vi "FTW-JSON-Serialize.vi"(0 "JSON Object":refnum<class "FTW-JSON.lvclass">, 11 "error in":errorcluster) -> (4 "JSON Object out":refnum<class "FTW-JSON.lvclass">, 6 "JSON String (UTF-8)":string, 15 "error out":errorcluster)   [LabVIEW 2012, in "FTW-JSON.lvclass"]
uses:
  FTW-JSON.lvclass
  FTW-JSON.lvclass/FTW-JSON.ctl
panel:
  # "Inputs"
  # "Outputs"
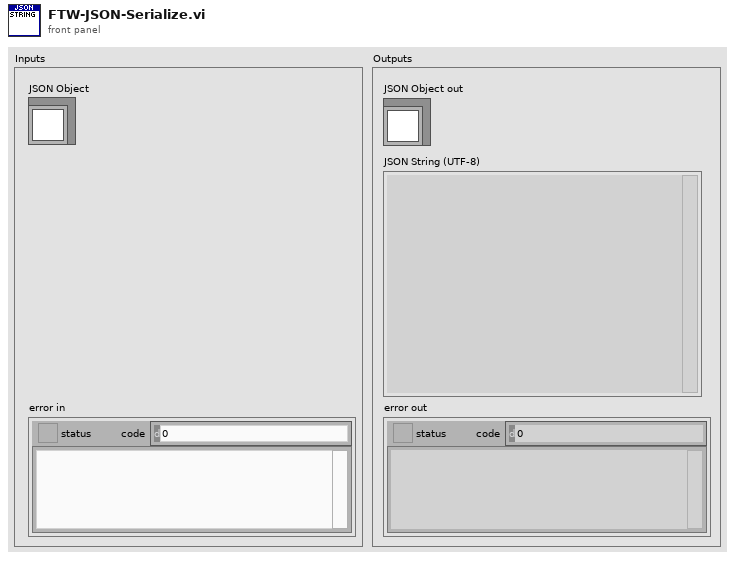
[diagram p1: front panel]
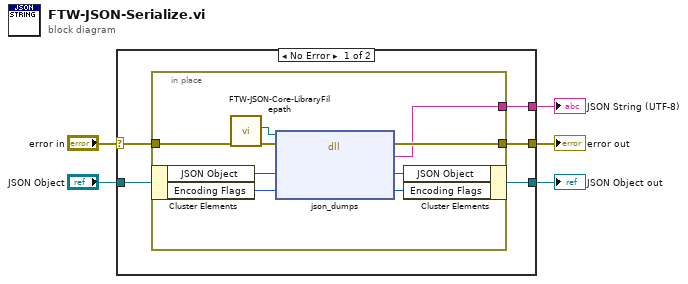
[diagram p0: block diagram]
diagram:
  n1 = case shown="No Error" "error in" {
    selector: "error in" -> [w10 w21]
    tunnel: [w9 w21] -> w5
    tunnel: [w7 w20] -> w3
    tunnel: "JSON Object" -> [w8 w20]
    tunnel: [w6 _] -> w1
    frame No Error {
      n2 = in-place {
        in-place-border: w10 -> [w19]
        in-place-border: [w16] -> w9
        in-place-border: [w13] -> w6
        n3 = in-place-cluster #1(w8) -> ("JSON Object"=w15:i64, "Encoding Flags"=w12:i64)
        n4 = call "FTW-JSON-Core-LibraryFilepath.vi"("error in"=w19) -> ("error out"=w18:errorcluster, "JSON Library Filepath"=w17:path)  [unwired: 9 in]
        n5 = dll-call lib="?" fn="json_dumps"(path in=w17, error in=w18, "JSON Object Pointer"=w15, "Flags"=w12) -> (error out=w16:errorcluster, "JSON String"=w13:string, "JSON Object Pointer"=w14:i64, "Flags"=w11:i64)  [unwired: 1 in, 1 out]
        n6 = in-place-cluster #1("JSON Object"=w14, "Encoding Flags"=w11) -> (w7:refnum<class "FTW-JSON.lvclass">)
      }
    }
    frame Error {
    }
  }
  "error out" <- w5
  "JSON Object out" <- w3
  "JSON String (UTF-8)" <- w1
